vi "c_ctre_phoenix6_platform_replay_is_running.vi"(0 "Numeric":u8, 1 "Numeric 2":u16) -> ()   [LabVIEW 2023]
uses:
  <vilib>/Rock Robotics/WPI/ThirdParty/Phoenix-LabVIEW/Controls/DriverLib.ctl
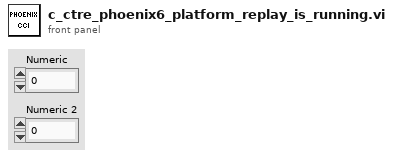
[diagram p1: front panel]
types:
  T1 = typedef "DriverLib.ctl" = path
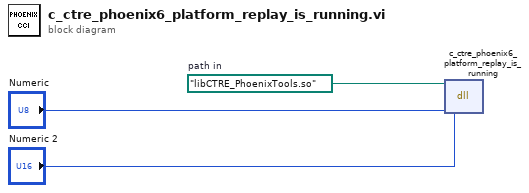
[diagram p0: block diagram]
diagram:
  w3 = T1 path "libCTRE_PhoenixTools.so"  # path in
  n1 = dll-call lib="?" fn="c_ctre_phoenix6_platform_replay_is_running"(path in=w3, "Numeric", "Numeric 2") -> ()  [unwired: 3 in, 2 out]
